vi "NewTPC.vi"(11 "Tab Control":enum32{"Page 1"}(tab)) -> ()   [LabVIEW 2023]
uses:
  <vilib>/Utility/file.llb/Read Delimited Spreadsheet (DBL).vi
panel:
  out "RowSize":i32
  out "all rows 2 - hiden":dbl[][](array[numeric])
  out "Stds by row in results":dbl[][](graph)
  out "Numeric":i32
  out "String":string
  out "Official result":dbl[](array[numeric])
  out "Current row":i64[](array[numeric])
  out "XY Graph":cluster{i32[], "Last official draw":i64[]}[](graph)
  out "Blincking":bool
  in  "Rows":u64
  in  "Cancel":bool
  in  "DEV":bool
  in  "Play":bool
  out "Last Suppose":dbl[][](graph)
  out "6@49":dbl[][](graph)
  out "Last Draw":i64[](array[numeric])
  out "Deviation":T1
  out "Data":T2
  out "STD":T3 {"STD 6@49" format="%#_4g"; "STD Last Suppose" format="%#_4g"; "STD Last Draw" format="%#_4g"}
  out "appended array":string[](array[string])
  out "Invisible tmp arr":dbl[][](array[numeric])
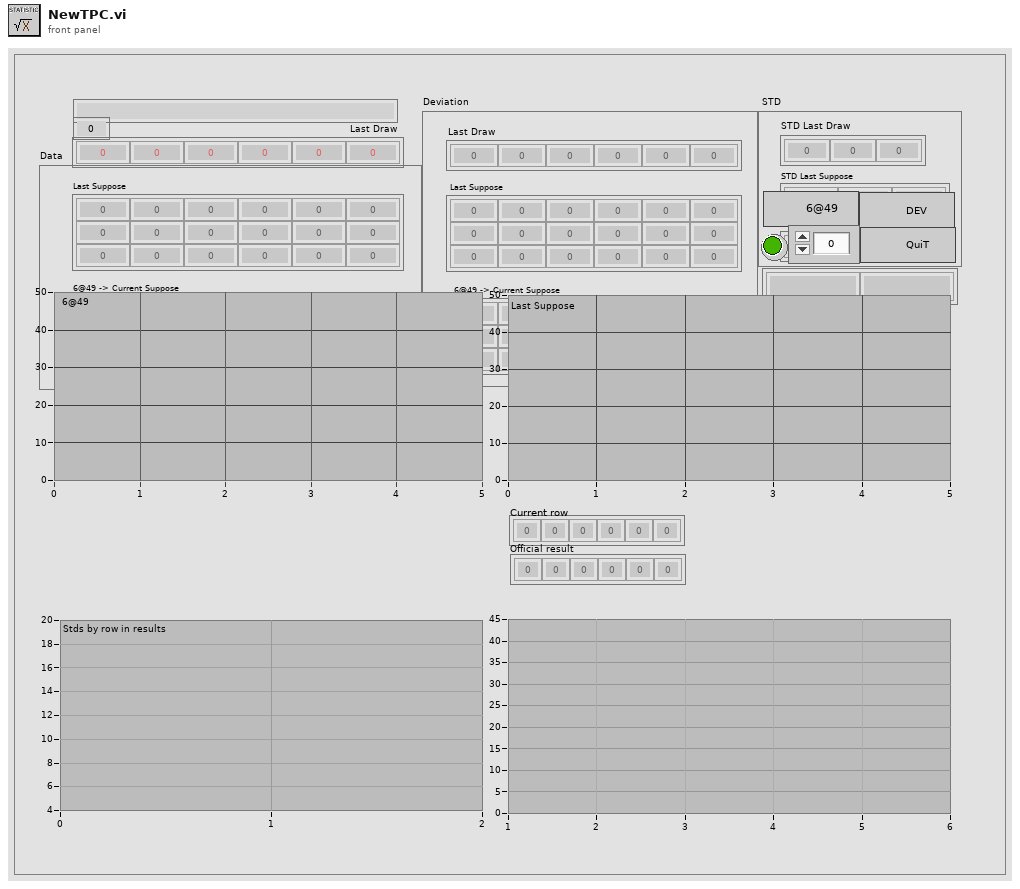
[diagram p1: front panel]
types:
  T1 = cluster{"Last Draw":i64[][], "Last Suppose":i64[][], "6@49 -> Current Suppose":i64[][]}
  T2 = cluster{"Last Suppose":i64[][], "6@49 -> Current Suppose":i64[][]}
  T3 = cluster{"STD Last Draw":dbl[], "STD Last Suppose":dbl[], "STD 6@49":dbl[]}
  T4 = cluster{"1D Std":dbl[], "1D Std":dbl[], "1D Std":dbl[]}
  T5 = cluster{"[Xi-X]":dbl[][], "[Xi-X]":dbl[][], "[Xi-X]":dbl[][]}
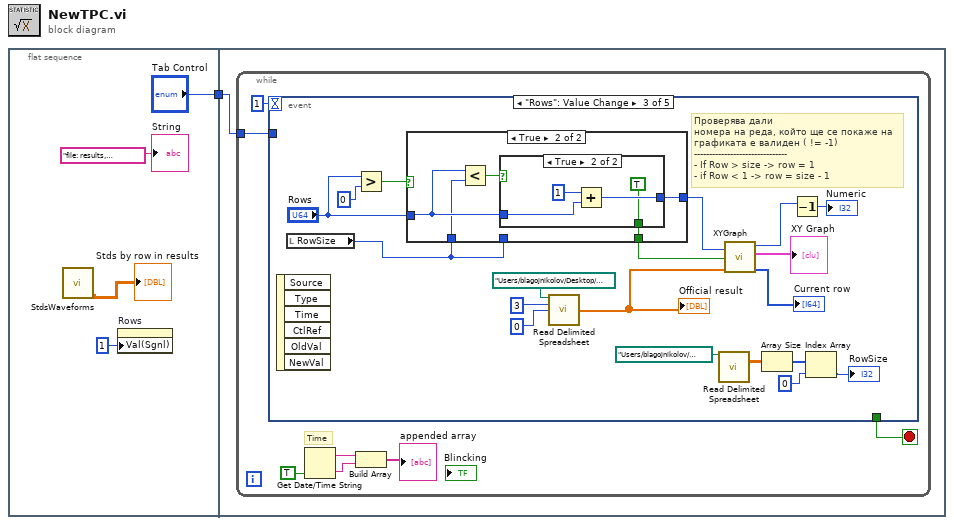
[diagram p0: block diagram]
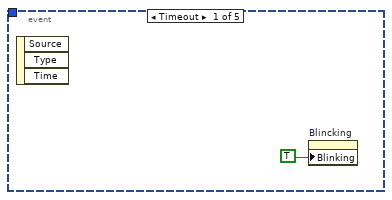
[diagram p2: hidden frame]
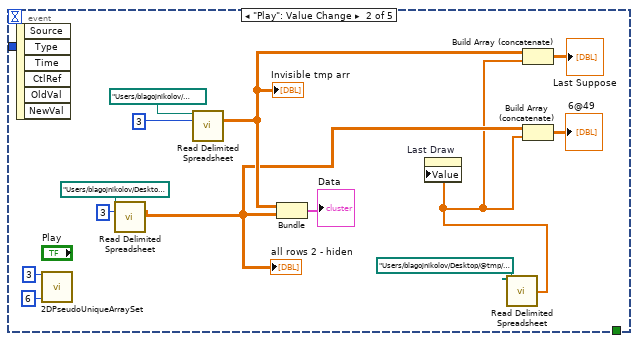
[diagram p3: hidden frame]
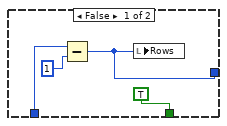
[diagram p4: hidden frame]
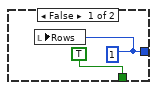
[diagram p5: hidden frame]
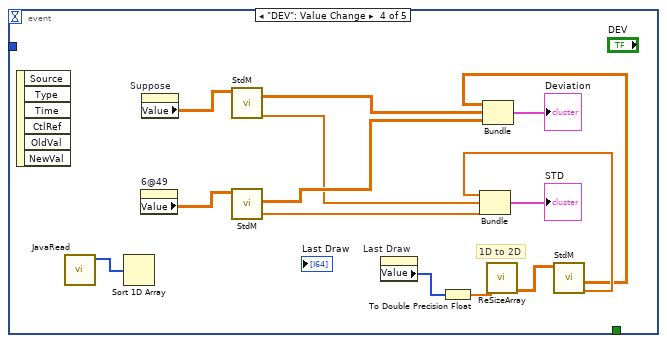
[diagram p6: hidden frame]
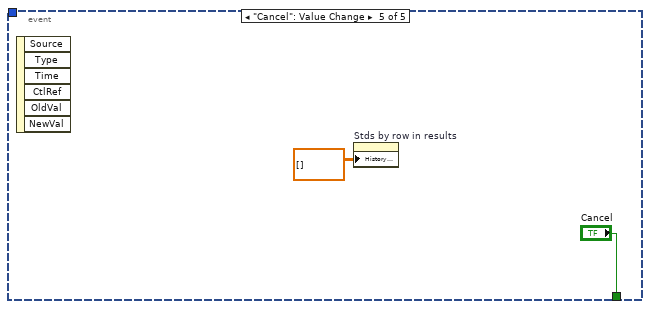
[diagram p7: hidden frame]
diagram:
  n1 = flat-sequence {
    tunnel: ["Tab Control"] -> w1
    tunnel: w1 -> [w6]
    frame #0 {
      n2 = call "StdsWaveforms.vi"() -> ("Std 1D Array"=→"Stds by row in results":dbl[][])  [unwired: 9 in, 2 out]
      n3 = property on="Rows" class="DigNum (strict)"("Val(Sgnl)"=u64 1 ("Value (Signaling)")) -> ()  [unwired: 2 in, 2 out]
      "String" <- "file: results, officialResults, checkRes, tmp649Gen.txt    " ("String")
    }
    frame #1 {
      n4 = while {
        tunnel: w6 -> [w13]
        stop <- w12 stop-if-true
        # "Time"
        n5 = event shown="[2] \"Rows\": Value Change" {
          selector: _ -> [_ _ _ _ _]
          dyn-events: _ -> [_ _ _ _ _]
          timeout: 1 -> [_ _ _ _ _]
          tunnel: w13 -> [_ _ _ _ _]
          tunnel: [_ _ _ _ "Cancel"] -> w12
          event Timeout {
            n6 = event-data() -> ()  [unwired: 1 in, 3 out]
            n7 = property on="Blincking" class="Bool (strict)"("Blinking"=TRUE) -> ()  [unwired: 2 in, 2 out]
          }
          event "Play": Value Change {
            n8 = event-data() -> ()  [unwired: 1 in, 6 out]
            n9 = call "2DPseudoUniqueArraySet.vi"("Colums"=6, "Rows"=3) -> ()  [unwired: 8 in, 2 out]
            n10 = call-poly <vilib>:"Read Delimited Spreadsheet.vi"("file path (dialog if empty)"=path "/Users/blagojnikolov/Desktop/@tmp/tmp649Gen.txt", "number of rows (all:-1)"=3 ("max characters/row  (no limit:0)")) -> ("all rows"=w17:dbl[][])  [unwired: 8 in, 5 out]
            "all rows 2 - hiden" <- w17
            n11 = call-poly <vilib>:"Read Delimited Spreadsheet.vi"("file path (dialog if empty)"=path "/Users/blagojnikolov/Desktop/@tmp/checkRes.txt", "number of rows (all:-1)"=3 ("max characters/row  (no limit:0)")) -> ("all rows"=w24:dbl[][])  [unwired: 8 in, 5 out]
            "Invisible tmp arr" <- w24
            n12 = Bundle("all rows"=w24, "all rows"=w17) -> (→"Data":cluster{"all rows":dbl[][], "all rows":dbl[][]})  [unwired: 1 in]
            n13 = call-poly <vilib>:"Read Delimited Spreadsheet.vi"("file path (dialog if empty)"=path "/Users/blagojnikolov/Desktop/@tmp/officialResults.txt") -> ("first row"=w15:dbl[])  [unwired: 9 in, 5 out]
            n14 = property on="Last Draw" class="Arr (strict)"("Value"=w15) -> ()  [unwired: 2 in, 2 out]
            n15 = Build Array (concatenate)(w24, w15) -> (→"Last Suppose":dbl[][])
            n16 = Build Array (concatenate)(w17, w15) -> (→"6@49":dbl[][])
          }
          event "Rows": Value Change {
            # "Проверява дали\nномера на реда, който ще се покаже на графиката е валиден ( != -1)\n-------------------------------\n- If Row > size -> row = 1 \n- if Row < 1 -> row = size - 1"
            n17 = event-data() -> ()  [unwired: 1 in, 6 out]
            n18 = local read "RowSize"() -> (w28:i32)
            n19 = Greater?(x="Rows", y=u64 0) -> (0:w39:bool)
            n20 = case shown="True" w39 {
              tunnel: [w49 w55] -> w42
              tunnel: "Rows" -> [_ w53]
              tunnel: [TRUE w54] -> w41
              tunnel: w28 -> [w48 _]
              tunnel: w28 -> [_ w51]
              frame False {
                n21 = Subtract(x=w48, y=1 ("x")) -> (x-y=w49:i32)
                n22 = local write "Rows"(w49) -> ()
              }
              frame True {
                n23 = Less?(x=w53, y=w51) -> (x < y?=w52:bool)
                n24 = case shown="True" w52 {
                  tunnel: [w56 w60] -> w55
                  tunnel: w53 -> [_ w59]
                  tunnel: [TRUE TRUE] -> w54
                  frame False {
                    w56 = u64 1
                    n25 = local write "Rows"(w56) -> ()
                  }
                  frame True {
                    n26 = Add(x=u64 1, y=w59) -> (x+y=w60:u64)
                  }
                }
              }
            }
            n27 = call-poly <vilib>:"Read Delimited Spreadsheet.vi"("file path (dialog if empty)"=path "/Users/blagojnikolov/Desktop/@tmp/officialResults.txt", "number of rows (all:-1)"=3 ("max characters/row  (no limit:0)"), "start of read offset (chars.:0)"=0) -> ("first row"=w34:dbl[])  [unwired: 7 in, 5 out]
            "Official result" <- w34
            n28 = call-poly <vilib>:"Read Delimited Spreadsheet.vi"("file path (dialog if empty)"=path "/Users/blagojnikolov/Desktop/@tmp/fromSite.txt") -> ("all rows"=w32:dbl[][])  [unwired: 9 in, 5 out]
            n29 = call "XYGraph.vi"("Last official draw"=w34, "stop"=w41, "Row"=w42) -> ("This row"=→"Current row":i64[], "Appended array"=→"XY Graph":cluster{i32[], "Last official draw":i64[]}[], "Draw Num"=w36:i32)  [unwired: 5 in, 1 out]
            n30 = Array Size(array=w32) -> (size(s)=w31:i32[])
            n31 = Decrement(x=w36) -> (x-1=→"Numeric":i32)
            n32 = Index Array(array=w31, index=0) -> (element=→"RowSize":i32)
          }
          event "DEV": Value Change {
            # "1D to 2D"
            n33 = event-data() -> ()  [unwired: 1 in, 6 out]
            n34 = call "JavaRead.vi"() -> ("First line"=w73:i64[])  [unwired: 10 in, 1 out]
            n35 = Sort 1D Array(array=w73) -> ()  [unwired: 1 out]
            n36 = property on="6@49" class="Arr (strict)"() -> ("Value"=w70:dbl[][])  [unwired: 2 in, 2 out]
            n37 = property on="Suppose" class="Arr (strict)"() -> ("Value"=w67:dbl[][])  [unwired: 2 in, 2 out]
            n38 = call "StdM.vi"("2D"=w67) -> ("1D Std"=w69:dbl[], "[Xi-X]"=w68:dbl[][])  [unwired: 6 in, 3 out]
            n39 = call "StdM.vi"("2D"=w70) -> ("1D Std"=w72:dbl[], "[Xi-X]"=w71:dbl[][])  [unwired: 6 in, 3 out]
            n40 = property on="Last Draw" class="Arr (strict)"() -> ("Value"=w63:i64[])  [unwired: 2 in, 2 out]
            n41 = To Double Precision Float(number=w63) -> (double precision float=w62:dbl[])
            n42 = call "ReSizeArray.vi"("1D"=w62) -> ("2D"=w64:dbl[][])  [unwired: 9 in, 1 out]
            n43 = call "StdM.vi"("2D"=w64) -> ("1D Std"=w66:dbl[], "[Xi-X]"=w65:dbl[][])  [unwired: 6 in, 3 out]
            n44 = Bundle("1D Std"=w66, "1D Std"=w69, "1D Std"=w72) -> (→"STD":T4)  [unwired: 1 in]
            n45 = Bundle "Bundle"("[Xi-X]"=w65, "[Xi-X]"=w68, "[Xi-X]"=w71) -> (→"Deviation":T5)  [unwired: 1 in]
          }
          event "Cancel": Value Change {
            n46 = event-data() -> ()  [unwired: 1 in, 6 out]
            n47 = property on="Stds by row in results" class="WFChart (strict)"("History Data"=dbl[][] []) -> ()  [unwired: 2 in, 2 out]
          }
        }
        n48 = Get Date/Time String(want seconds? (F)=TRUE) -> (date string=w10:string, time string=w9:string)  [unwired: 2 in]
        n49 = Build Array(w10, w9) -> (→"appended array":string[])
      }
    }
  }
